vi "Example OpenCV Object Tracking3.0.vi"() -> ()   [LabVIEW 2014]
uses:
  vi.lib/Q-WaveSystems/QwaveSys Raspberry Pi for LabVIEW Home-Education/QwaveSys Raspberry Pi Library.lvlib
panel:
  in  "Upper (SV)":i32(slide)=223 scale=0.0..255.0
  in  "Lower (SV)":i32(slide)=58 scale=0.0..255.0
  out "H-H":u8=111
  out "L-H":u8=105
  out "Color Box Upper":u32=16860
  out "Color Box Lower":u32=3381759
  in  "Fine Tune Upper":i32(slide)=119 scale=91.0..131.0
  in  "Fine Tune  Lower":i32(slide)=98 scale=85.0..125.0
  in  "Color Upper":u32(colorbox)=16860
  in  "Color Lower":u32(colorbox)=3381759
  out "XYR found":u32[][](array[numeric])=[[183, 192, 10]]
  in  "Max_radius":i32(slide)=50 scale=0.0..100.0
  in  "Min_radius":i32(slide)=7 scale=0.0..100.0
  out "found":i32=1
  in  "webcamnum":i32
  in  "STOP":bool caption="Blank Button"
  # "H"
  # "H"
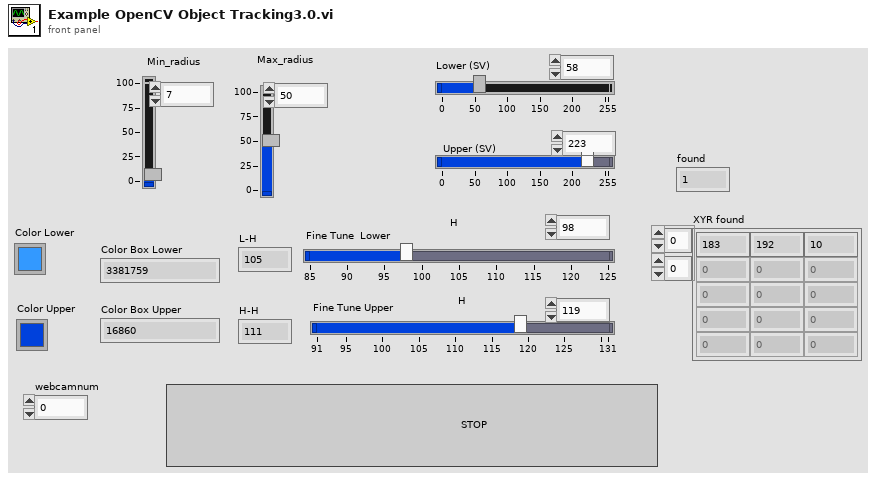
[diagram p1: front panel]
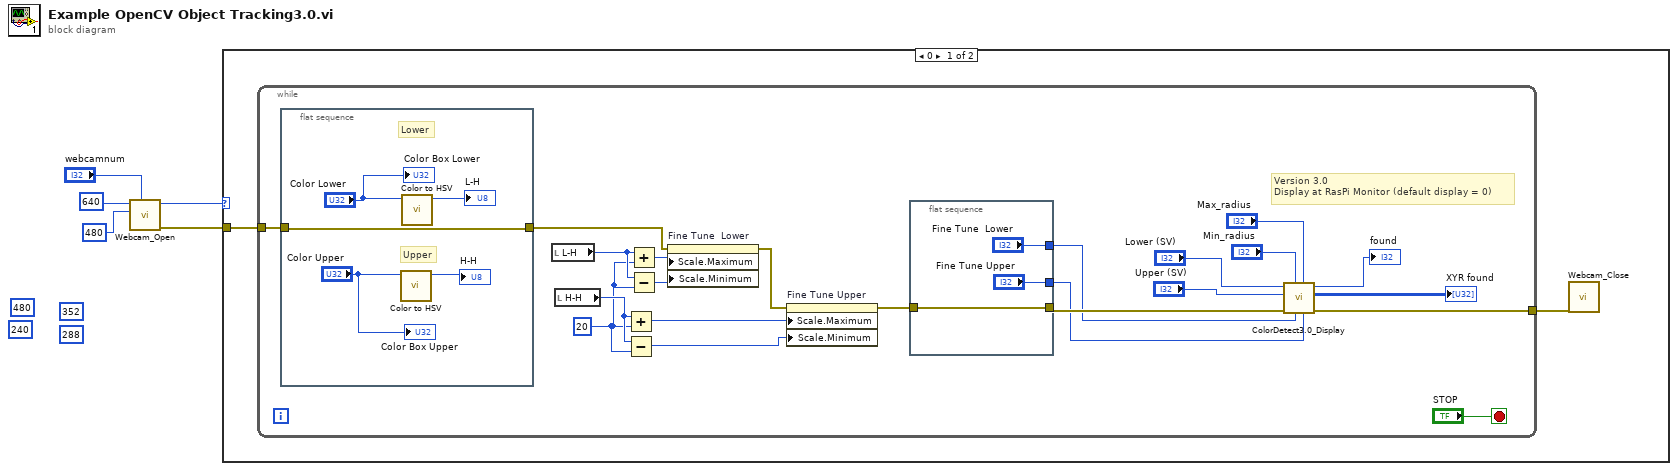
[diagram p0: block diagram]
diagram:
  (unwired) u32 288 ("height")
  (unwired) u32 352 ("width")
  (unwired) u32 240 ("height")
  (unwired) u32 480 ("width")
  n1 = call "Webcam_Open.vi"("webcamnum"="webcamnum", "height"=u32 480, "width"=u32 640) -> ("error out"=w3:errorcluster, "return type"=w2:i32)  [unwired: 7 in]
  n2 = case shown="0" w2 {
    tunnel: w3 -> [w7 _]
    frame 0 {
      n3 = while {
        tunnel: w7 -> [w19]
        tunnel: [w16] -> w6
        stop <- "STOP" stop-if-true
        w22 = 20 ("y")
        # "Version 3.0\nDisplay at RasPi Monitor (default display = 0)"
        n4 = flat-sequence {
          tunnel: w19 -> [w30]
          tunnel: [w30] -> w18
          frame #0 {
            # "Upper"
            # "Lower"
            n5 = call "Color to HSV.vi"("Color Box"="Color Upper") -> ("Hue (0-180)"=→"H-H":u8)  [unwired: 8 in, 2 out]
            n6 = call "Color to HSV.vi"("Color Box"="Color Lower") -> ("Hue (0-180)"=→"L-H":u8)  [unwired: 8 in, 2 out]
            "Color Box Upper" <- "Color Upper"
            "Color Box Lower" <- "Color Lower"
          }
        }
        n7 = local read "L-H"() -> (w23:u8)
        n8 = local read "H-H"() -> (w27:u8)
        n9 = Add(x=w27, y=w22) -> (x+y=w28:i32)
        n10 = Subtract(x=w27, y=w22) -> (x-y=w26:i32)
        n11 = Add(x=w23, y=w22) -> (x+y=w25:i32)
        n12 = Subtract(x=w23, y=w22) -> (x-y=w24:i32)
        n13 = property on="Fine Tune  Lower" class="Slide (strict)"(error in=w18, "Scale.Maximum"=w25, "Scale.Minimum"=w24) -> (error out=w21:errorcluster)  [unwired: 1 in, 1 out]
        n14 = property on="Fine Tune Upper" class="Slide (strict)"(error in=w21, "Scale.Maximum"=w28, "Scale.Minimum"=w26) -> (error out=w20:errorcluster)  [unwired: 1 in, 1 out]
        n15 = flat-sequence {
          tunnel: [w37] -> w17
          tunnel: w20 -> [w37]
          tunnel: ["Fine Tune  Lower"] -> w11
          tunnel: ["Fine Tune Upper"] -> w10
          frame #0 {
          }
        }
        n16 = call "ColorDetect3.0_Display.vi"("Fine Tune Upper"=w10, "Max_radius"="Max_radius", "Fine Tune  Lower"=w11, "Min_radius"="Min_radius", "error in (no error)"=w17, "Upper (SV)"="Upper (SV)", "Lower (SV)"="Lower (SV)") -> ("error out"=w16:errorcluster, "XYR found"=→"XYR found":u32[][], "found"=→"found":i32)  [unwired: 2 in]
      }
      n17 = call "Webcam_Close.vi"("error in (no error)"=w6) -> ()  [unwired: 10 in, 1 out]
    }
    frame -1, Default {
      # "No Camera Found"
    }
  }
